vi "UpdateAttribute.vi"(8 "error in (no error)":errorcluster, 9 "Attribute Name":string, 10 "Attribute":refnum<class "Attribute.lvclass">, 11 "SMO in":refnum<class "SMO.lvclass">) -> (0 "error out":errorcluster, 2 "replaced":bool, 3 "SMO out":refnum<class "SMO.lvclass">)   [LabVIEW 2013, in "SMO.lvclass"]
uses:
  SMO.lvclass
  Support/Attribute/Attribute.lvclass
  SMO.lvclass/SMO.ctl
  Support/Attribute/Attribute.lvclass/Attribute.ctl
  <vilib>/Utility/LVClass/Get LV Class Name.vi
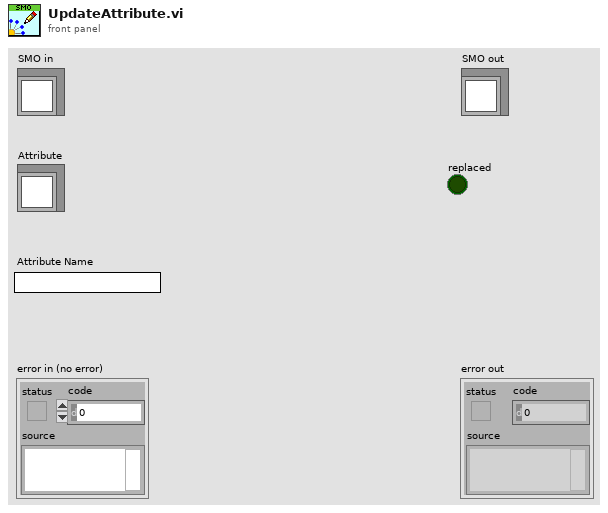
[diagram p1: front panel]
types:
  T1 = typedef "SMO.lvclass/PrivateData--Ref.ctl" = refnum<data-value>
  T2 = typedef "SMO.lvclass/PrivateData--Cluster.ctl" = cluster{"Parent Call":T3, "Registered Processes":T4[], "Sync Notifier":refnum<notifier>, "Process Error Notifier":refnum<notifier>, "Protected Events":T5, "Public Events":T6, "SMO State":T7, "[Attributes]":variant, "Launcher Close":refnum<notifier>, "Caller Watchdog":refnum<queue>, "Accessibility":T8, "NbStaticDependencies":u32}
  T3 = typedef "SMO.lvclass/Parent Call--Enum.ctl" = enum16{"Allows parent to run", "Does not request parent to run"}
  T4 = typedef "SMO.lvclass/RegisteredProcessData--Cluster.ctl" = cluster{"Name":string, "Static VI Ref":refnum<vi>, "Running":bool, "NotifierRef":u32}
  T5 = typedef "SMO.lvclass/Protected Events.ctl" = cluster{"StopProcesses":refnum<user-event>, "AbortProcesses":refnum<user-event>, "Config Changed":refnum<user-event>, "Dependency":refnum<user-event>}
  T6 = typedef "SMO.lvclass/Public Events.ctl" = cluster{"Error":refnum<user-event>, "State":refnum<user-event>, "Reserve State":refnum<user-event>}
  T7 = typedef "SMO.lvclass/SMOState --Enum.ctl" = enum16{"unknown", "Created", "Started", "Stopped"}
  T8 = typedef "SMO.lvclass/Accessibility--Cluster.ctl" = cluster{"Lock Key":string, "Reserve State":T9}
  T9 = typedef "SMO.lvclass/Reserve State--Enum.ctl" = enum16{"Unreserved", "Reserved", "Self-locked"}
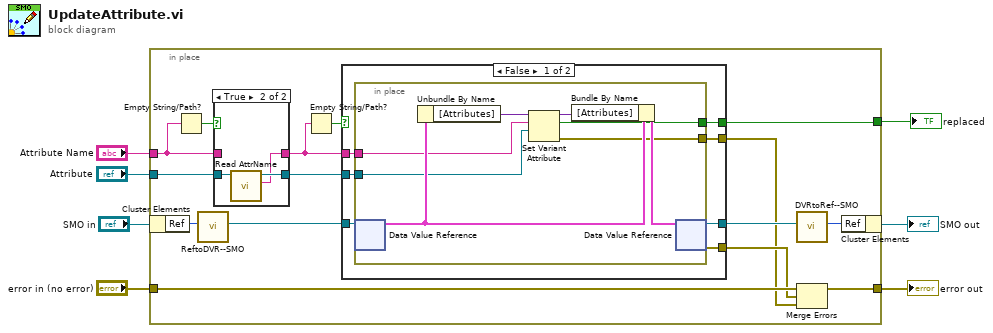
[diagram p0: block diagram]
diagram:
  n1 = in-place {
    in-place-border: "error in (no error)" -> [w18]
    in-place-border: [w16] -> w4
    in-place-border: "Attribute" -> [w12]
    in-place-border: "Attribute Name" -> [w13]
    in-place-border: [w8] -> w1
    n2 = in-place-cluster #1("SMO in") -> ("Ref"=w22:u32)
    n3 = Empty String/Path?(string/path=w13) -> (empty?=w14:bool)
    n4 = call "ReftoDVR--SMO.vi"("Ref"=w22) -> ("Ref"=w21:T1)  [unwired: 10 in]
    n5 = case shown="True" w14 {
      tunnel: w13 -> [w40 _]
      tunnel: [w40 w41] -> w10
      tunnel: w12 -> [w39 w43]
      tunnel: [w39 w42] -> w11
      frame False {
      }
      frame True {
        n6 = call "Read AttrName.vi"("Attribute in"=w43) -> ("Attribute Name"=w41:string, "Attribute out"=w42:refnum<class "Attribute.lvclass">)  [unwired: 9 in]
      }
    }
    n7 = Empty String/Path?(string/path=w10) -> (empty?=w9:bool)
    n8 = case shown="False" w9 {
      tunnel: w21 -> [w29 w38]
      tunnel: [w28 w38] -> w20
      tunnel: [w27 _] -> w17
      tunnel: [w26 _] -> w15
      tunnel: w11 -> [w25 _]
      tunnel: w10 -> [w24 _]
      tunnel: [w23 _] -> w8
      frame False {
        n9 = in-place {
          in-place-border: w25 -> [w32]
          in-place-border: w24 -> [w33]
          in-place-border: [w31] -> w26
          in-place-border: [w30] -> w23
          n10 = in-place-dvr #2(w29) -> (w36:T2)  [unwired: 1 out]
          n11 = Unbundle By Name(w36) -> ("[Attributes]"=w35:variant)
          n12 = Set Variant Attribute(Variant=w35, name=w33, value=w32) -> (Variant out=w34:variant, replaced=w30:bool, error out=w31:errorcluster)  [unwired: 1 in]
          n13 = Bundle By Name(cluster=w36, "[Attributes]"=w34) -> (w37:T2)
          n14 = in-place-dvr #2(w37) -> (w28:T1, w27:errorcluster)
        }
      }
      frame True {
      }
    }
    n15 = call "DVRtoRef--SMO.vi"("Ref"=w20) -> ("Ref"=w19:u32)  [unwired: 10 in]
    n16 = Merge Errors(w18, w17, w15) -> (w16:errorcluster)
    n17 = in-place-cluster #1("Ref"=w19) -> (→"SMO out":refnum<class "SMO.lvclass">)
  }
  "error out" <- w4
  "replaced" <- w1
